vi "ConvertEdgesToLines.vi"(8 "HomeXY(pixels)":cluster{dbl, dbl}, 9 "PixelmmRatio":dbl format="%#_13g", 10 "Horizontal Edges":T1(array[cluster]) {"Point2 (Real-World)"."Y" format="%.2f"; "Point2 (Real-World)"."X" format="%.2f"; "Point1 (Real-World)"."Y" format="%.2f"; "Point1 (Real-World)"."X" format="%.2f"; "Point2 (Pixels)"."Y" format="%.2f"; "Point2 (Pixels)"."X" format="%.2f"; "Point1 (Pixels)"."Y" format="%.2f"; "Point1 (Pixels)"."X" format="%.2f"}, 11 "Vertical Edges":T1(array[cluster]) {"Point2 (Real-World)"."Y" format="%.2f"; "Point2 (Real-World)"."X" format="%.2f"; "Point1 (Real-World)"."Y" format="%.2f"; "Point1 (Real-World)"."X" format="%.2f"; "Point2 (Pixels)"."Y" format="%.2f"; "Point2 (Pixels)"."X" format="%.2f"; "Point1 (Pixels)"."Y" format="%.2f"; "Point1 (Pixels)"."X" format="%.2f"}) -> (1 "Lw Right":dbl[](array[numeric]), 2 "Lw Left":dbl[](array[numeric]), 3 "Lg":dbl[](array[numeric]))   [LabVIEW 2017]
uses:
  <vilib>/vision/NI_Vision_Development_Module.lvlib
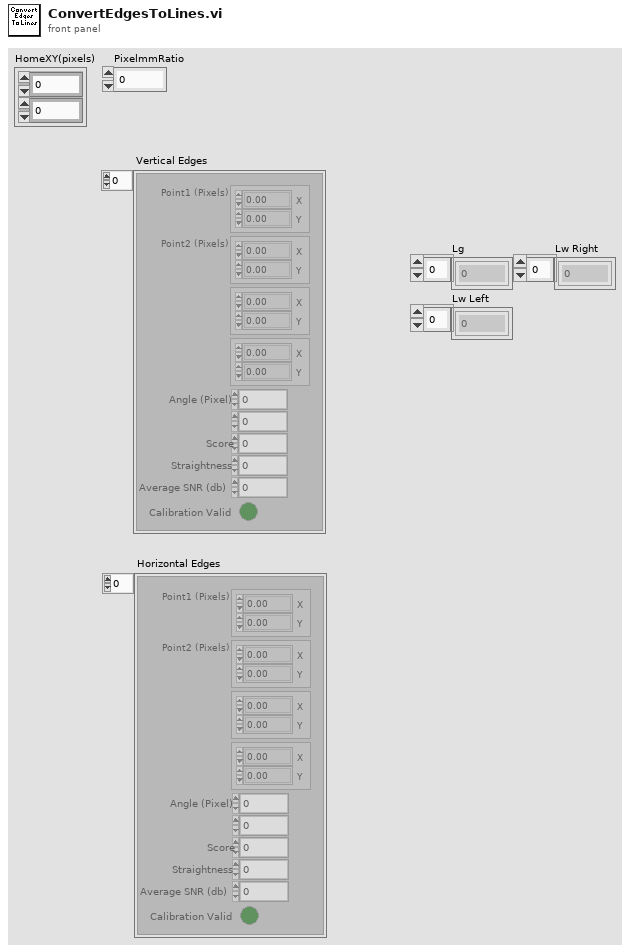
[diagram p1: front panel]
types:
  T1 = cluster{"Point1 (Pixels)":cluster{"X":sgl, "Y":sgl}, "Point2 (Pixels)":cluster{"X":sgl, "Y":sgl}, "Point1 (Real-World)":cluster{"X":sgl, "Y":sgl}, "Point2 (Real-World)":cluster{"X":sgl, "Y":sgl}, "Angle (Pixel)":dbl, "Angle (Real-World)":dbl, "Score":dbl, "Straightness":dbl, "Average SNR (db)":dbl, "Calibration Valid":bool}[]
  T2 = cluster{"Vertical Edges[0]":cluster{"Point1 (Pixels)":cluster{"X":sgl, "Y":sgl}, "Point2 (Pixels)":cluster{"X":sgl, "Y":sgl}, "Point1 (Real-World)":cluster{"X":sgl, "Y":sgl}, "Point2 (Real-World)":cluster{"X":sgl, "Y":sgl}, "Angle (Pixel)":dbl, "Angle (Real-World)":dbl, "Score":dbl, "Straightness":dbl, "Average SNR (db)":dbl, "Calibration Valid":bool}, "Vertical Edges[1]":cluster{"Point1 (Pixels)":cluster{"X":sgl, "Y":sgl}, "Point2 (Pixels)":cluster{"X":sgl, "Y":sgl}, "Point1 (Real-World)":cluster{"X":sgl, "Y":sgl}, "Point2 (Real-World)":cluster{"X":sgl, "Y":sgl}, "Angle (Pixel)":dbl, "Angle (Real-World)":dbl, "Score":dbl, "Straightness":dbl, "Average SNR (db)":dbl, "Calibration Valid":bool}, "Vertical Edges[2]":cluster{"Point1 (Pixels)":cluster{"X":sgl, "Y":sgl}, "Point2 (Pixels)":cluster{"X":sgl, "Y":sgl}, "Point1 (Real-World)":cluster{"X":sgl, "Y":sgl}, "Point2 (Real-World)":cluster{"X":sgl, "Y":sgl}, "Angle (Pixel)":dbl, "Angle (Real-World)":dbl, "Score":dbl, "Straightness":dbl, "Average SNR (db)":dbl, "Calibration Valid":bool}, "Vertical Edges[3]":cluster{"Point1 (Pixels)":cluster{"X":sgl, "Y":sgl}, "Point2 (Pixels)":cluster{"X":sgl, "Y":sgl}, "Point1 (Real-World)":cluster{"X":sgl, "Y":sgl}, "Point2 (Real-World)":cluster{"X":sgl, "Y":sgl}, "Angle (Pixel)":dbl, "Angle (Real-World)":dbl, "Score":dbl, "Straightness":dbl, "Average SNR (db)":dbl, "Calibration Valid":bool}, "Vertical Edges[4]":cluster{"Point1 (Pixels)":cluster{"X":sgl, "Y":sgl}, "Point2 (Pixels)":cluster{"X":sgl, "Y":sgl}, "Point1 (Real-World)":cluster{"X":sgl, "Y":sgl}, "Point2 (Real-World)":cluster{"X":sgl, "Y":sgl}, "Angle (Pixel)":dbl, "Angle (Real-World)":dbl, "Score":dbl, "Straightness":dbl, "Average SNR (db)":dbl, "Calibration Valid":bool}, "Vertical Edges[5]":cluster{"Point1 (Pixels)":cluster{"X":sgl, "Y":sgl}, "Point2 (Pixels)":cluster{"X":sgl, "Y":sgl}, "Point1 (Real-World)":cluster{"X":sgl, "Y":sgl}, "Point2 (Real-World)":cluster{"X":sgl, "Y":sgl}, "Angle (Pixel)":dbl, "Angle (Real-World)":dbl, "Score":dbl, "Straightness":dbl, "Average SNR (db)":dbl, "Calibration Valid":bool}, "Vertical Edges[6]":cluster{"Point1 (Pixels)":cluster{"X":sgl, "Y":sgl}, "Point2 (Pixels)":cluster{"X":sgl, "Y":sgl}, "Point1 (Real-World)":cluster{"X":sgl, "Y":sgl}, "Point2 (Real-World)":cluster{"X":sgl, "Y":sgl}, "Angle (Pixel)":dbl, "Angle (Real-World)":dbl, "Score":dbl, "Straightness":dbl, "Average SNR (db)":dbl, "Calibration Valid":bool}, "Vertical Edges[7]":cluster{"Point1 (Pixels)":cluster{"X":sgl, "Y":sgl}, "Point2 (Pixels)":cluster{"X":sgl, "Y":sgl}, "Point1 (Real-World)":cluster{"X":sgl, "Y":sgl}, "Point2 (Real-World)":cluster{"X":sgl, "Y":sgl}, "Angle (Pixel)":dbl, "Angle (Real-World)":dbl, "Score":dbl, "Straightness":dbl, "Average SNR (db)":dbl, "Calibration Valid":bool}, "Vertical Edges[8]":cluster{"Point1 (Pixels)":cluster{"X":sgl, "Y":sgl}, "Point2 (Pixels)":cluster{"X":sgl, "Y":sgl}, "Point1 (Real-World)":cluster{"X":sgl, "Y":sgl}, "Point2 (Real-World)":cluster{"X":sgl, "Y":sgl}, "Angle (Pixel)":dbl, "Angle (Real-World)":dbl, "Score":dbl, "Straightness":dbl, "Average SNR (db)":dbl, "Calibration Valid":bool}}
  T3 = cluster{"Horizontal Edges[0]":cluster{"Point1 (Pixels)":cluster{"X":sgl, "Y":sgl}, "Point2 (Pixels)":cluster{"X":sgl, "Y":sgl}, "Point1 (Real-World)":cluster{"X":sgl, "Y":sgl}, "Point2 (Real-World)":cluster{"X":sgl, "Y":sgl}, "Angle (Pixel)":dbl, "Angle (Real-World)":dbl, "Score":dbl, "Straightness":dbl, "Average SNR (db)":dbl, "Calibration Valid":bool}, "Horizontal Edges[1]":cluster{"Point1 (Pixels)":cluster{"X":sgl, "Y":sgl}, "Point2 (Pixels)":cluster{"X":sgl, "Y":sgl}, "Point1 (Real-World)":cluster{"X":sgl, "Y":sgl}, "Point2 (Real-World)":cluster{"X":sgl, "Y":sgl}, "Angle (Pixel)":dbl, "Angle (Real-World)":dbl, "Score":dbl, "Straightness":dbl, "Average SNR (db)":dbl, "Calibration Valid":bool}, "Horizontal Edges[2]":cluster{"Point1 (Pixels)":cluster{"X":sgl, "Y":sgl}, "Point2 (Pixels)":cluster{"X":sgl, "Y":sgl}, "Point1 (Real-World)":cluster{"X":sgl, "Y":sgl}, "Point2 (Real-World)":cluster{"X":sgl, "Y":sgl}, "Angle (Pixel)":dbl, "Angle (Real-World)":dbl, "Score":dbl, "Straightness":dbl, "Average SNR (db)":dbl, "Calibration Valid":bool}, "Horizontal Edges[3]":cluster{"Point1 (Pixels)":cluster{"X":sgl, "Y":sgl}, "Point2 (Pixels)":cluster{"X":sgl, "Y":sgl}, "Point1 (Real-World)":cluster{"X":sgl, "Y":sgl}, "Point2 (Real-World)":cluster{"X":sgl, "Y":sgl}, "Angle (Pixel)":dbl, "Angle (Real-World)":dbl, "Score":dbl, "Straightness":dbl, "Average SNR (db)":dbl, "Calibration Valid":bool}, "Horizontal Edges[4]":cluster{"Point1 (Pixels)":cluster{"X":sgl, "Y":sgl}, "Point2 (Pixels)":cluster{"X":sgl, "Y":sgl}, "Point1 (Real-World)":cluster{"X":sgl, "Y":sgl}, "Point2 (Real-World)":cluster{"X":sgl, "Y":sgl}, "Angle (Pixel)":dbl, "Angle (Real-World)":dbl, "Score":dbl, "Straightness":dbl, "Average SNR (db)":dbl, "Calibration Valid":bool}, "Horizontal Edges[5]":cluster{"Point1 (Pixels)":cluster{"X":sgl, "Y":sgl}, "Point2 (Pixels)":cluster{"X":sgl, "Y":sgl}, "Point1 (Real-World)":cluster{"X":sgl, "Y":sgl}, "Point2 (Real-World)":cluster{"X":sgl, "Y":sgl}, "Angle (Pixel)":dbl, "Angle (Real-World)":dbl, "Score":dbl, "Straightness":dbl, "Average SNR (db)":dbl, "Calibration Valid":bool}, "Horizontal Edges[6]":cluster{"Point1 (Pixels)":cluster{"X":sgl, "Y":sgl}, "Point2 (Pixels)":cluster{"X":sgl, "Y":sgl}, "Point1 (Real-World)":cluster{"X":sgl, "Y":sgl}, "Point2 (Real-World)":cluster{"X":sgl, "Y":sgl}, "Angle (Pixel)":dbl, "Angle (Real-World)":dbl, "Score":dbl, "Straightness":dbl, "Average SNR (db)":dbl, "Calibration Valid":bool}, "Horizontal Edges[7]":cluster{"Point1 (Pixels)":cluster{"X":sgl, "Y":sgl}, "Point2 (Pixels)":cluster{"X":sgl, "Y":sgl}, "Point1 (Real-World)":cluster{"X":sgl, "Y":sgl}, "Point2 (Real-World)":cluster{"X":sgl, "Y":sgl}, "Angle (Pixel)":dbl, "Angle (Real-World)":dbl, "Score":dbl, "Straightness":dbl, "Average SNR (db)":dbl, "Calibration Valid":bool}, "Horizontal Edges[8]":cluster{"Point1 (Pixels)":cluster{"X":sgl, "Y":sgl}, "Point2 (Pixels)":cluster{"X":sgl, "Y":sgl}, "Point1 (Real-World)":cluster{"X":sgl, "Y":sgl}, "Point2 (Real-World)":cluster{"X":sgl, "Y":sgl}, "Angle (Pixel)":dbl, "Angle (Real-World)":dbl, "Score":dbl, "Straightness":dbl, "Average SNR (db)":dbl, "Calibration Valid":bool}}
  T4 = cluster{"Point1 (Pixels)":cluster{"X":sgl, "Y":sgl}, "Point2 (Pixels)":cluster{"X":sgl, "Y":sgl}, "Point1 (Real-World)":cluster{"X":sgl, "Y":sgl}, "Point2 (Real-World)":cluster{"X":sgl, "Y":sgl}, "Angle (Pixel)":dbl, "Angle (Real-World)":dbl, "Score":dbl, "Straightness":dbl, "Average SNR (db)":dbl, "Calibration Valid":bool}
  T5 = cluster{"Point1 (Real-World)":cluster{"X":sgl, "Y":sgl}, "Point2 (Real-World)":cluster{"X":sgl, "Y":sgl}}
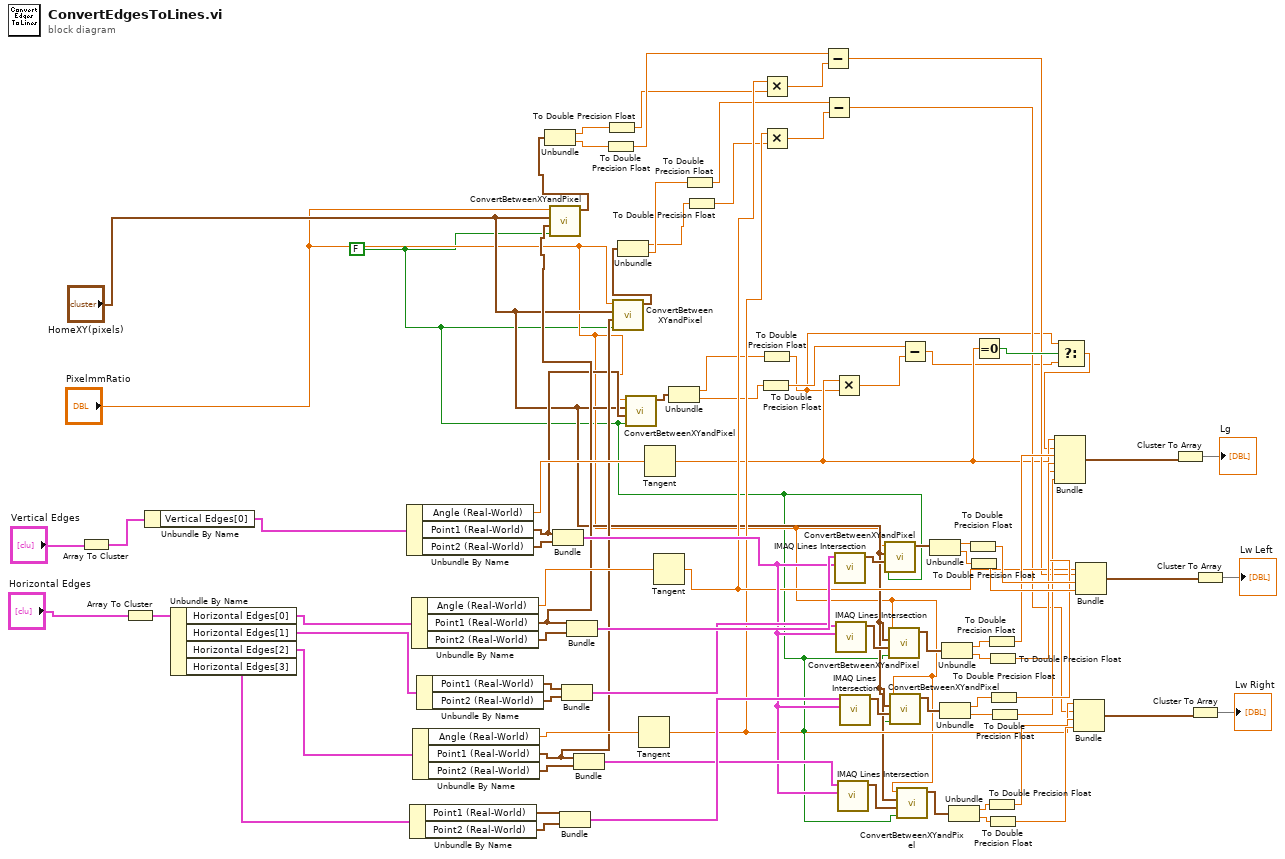
[diagram p0: block diagram]
diagram:
  w1 = FALSE ("XYtoPixels")
  n1 = Array To Cluster(array="Vertical Edges") -> (cluster=w85:T2)
  n2 = Array To Cluster(array="Horizontal Edges") -> (cluster=w83:T3)
  n3 = Unbundle By Name(w85) -> ("Vertical Edges[0]"=w77:T4)
  n4 = Unbundle By Name(w83) -> ("Horizontal Edges[0]"=w82:T4, "Horizontal Edges[1]"=w79:T4, "Horizontal Edges[2]"=w80:T4, "Horizontal Edges[3]"=w78:T4)
  n5 = Unbundle By Name(w77) -> ("Angle (Real-World)"=w68:dbl, "Point1 (Real-World)"=w7:cluster{"X":sgl, "Y":sgl}, "Point2 (Real-World)"=w75:cluster{"X":sgl, "Y":sgl})
  n6 = Unbundle By Name(w78) -> ("Point1 (Real-World)"=w72:cluster{"X":sgl, "Y":sgl}, "Point2 (Real-World)"=w71:cluster{"X":sgl, "Y":sgl})
  n7 = Unbundle By Name(w82) -> ("Angle (Real-World)"=w69:dbl, "Point1 (Real-World)"=w31:cluster{"X":sgl, "Y":sgl}, "Point2 (Real-World)"=w81:cluster{"X":sgl, "Y":sgl})
  n8 = Unbundle By Name(w80) -> ("Angle (Real-World)"=w70:dbl, "Point1 (Real-World)"=w27:cluster{"X":sgl, "Y":sgl}, "Point2 (Real-World)"=w76:cluster{"X":sgl, "Y":sgl})
  n9 = Unbundle By Name(w79) -> ("Point1 (Real-World)"=w74:cluster{"X":sgl, "Y":sgl}, "Point2 (Real-World)"=w73:cluster{"X":sgl, "Y":sgl})
  n10 = call "ConvertBetweenXYandPixel.vi"("XYtoPixels"=w1, "PointToConvert"=w31, "HomeXY(pixels)"="HomeXY(pixels)", "Pixel/mm"="PixelmmRatio") -> ("Point"=w30:cluster{sgl, sgl})  [unwired: 7 in]
  n11 = Unbundle(w30) -> (w29:sgl, w28:sgl)
  n12 = Bundle("Point1 (Real-World)"=w7, "Point2 (Real-World)"=w75) -> (w61:T5)  [unwired: 1 in]
  n13 = Bundle("Point1 (Real-World)"=w72, "Point2 (Real-World)"=w71) -> (w63:T5)  [unwired: 1 in]
  n14 = Bundle("Point1 (Real-World)"=w74, "Point2 (Real-World)"=w73) -> (w64:T5)  [unwired: 1 in]
  n15 = Bundle("Point1 (Real-World)"=w31, "Point2 (Real-World)"=w81) -> (w67:T5)  [unwired: 1 in]
  n16 = Bundle("Point1 (Real-World)"=w27, "Point2 (Real-World)"=w76) -> (w62:T5)  [unwired: 1 in]
  n17 = To Double Precision Float(number=w28) -> (double precision float=w49:dbl)
  n18 = To Double Precision Float(number=w29) -> (double precision float=w47:dbl)
  n19 = call "ConvertBetweenXYandPixel.vi"("XYtoPixels"=w1, "PointToConvert"=w27, "HomeXY(pixels)"="HomeXY(pixels)", "Pixel/mm"="PixelmmRatio") -> ("Point"=w26:cluster{sgl, sgl})  [unwired: 7 in]
  n20 = Unbundle(w26) -> (w24:sgl, w25:sgl)
  n21 = call "ConvertBetweenXYandPixel.vi"("XYtoPixels"=w1, "PointToConvert"=w7, "HomeXY(pixels)"="HomeXY(pixels)", "Pixel/mm"="PixelmmRatio") -> ("Point"=w6:cluster{sgl, sgl})  [unwired: 7 in]
  n22 = Tangent(1:w70) -> (0:w52:dbl)
  n23 = Tangent(1:w68) -> (0:w36:dbl)
  n24 = Tangent(1:w69) -> (0:w53:dbl)
  n25 = Unbundle(w6) -> (w5:sgl, w4:sgl)
  n26 = To Double Precision Float(number=w25) -> (double precision float=w48:dbl)
  n27 = To Double Precision Float(number=w24) -> (double precision float=w46:dbl)
  n28 = To Double Precision Float(number=w4) -> (double precision float=w45:dbl)
  n29 = Multiply(x=w53, y=w47) -> (x*y=w51:dbl)
  n30 = Multiply(x=w52, y=w46) -> (x*y=w50:dbl)
  n31 = To Double Precision Float(number=w5) -> (double precision float=w35:dbl)
  n32 = Subtract(x=w49, y=w51) -> (x-y=w38:dbl)
  n33 = Subtract(x=w48, y=w50) -> (x-y=w37:dbl)
  n34 = Multiply(x=w36, y=w35) -> (x*y=w44:dbl)
  n35 = call "IMAQ Lines Intersection"("Line 2"=w61, "Line 1"=w67) -> ("Intersection Point"=w20:cluster{"X":sgl, "Y":sgl})  [unwired: 7 in, 2 out]
  n36 = call "IMAQ Lines Intersection"("Line 2"=w61, "Line 1"=w64) -> ("Intersection Point"=w19:cluster{"X":sgl, "Y":sgl})  [unwired: 7 in, 2 out]
  n37 = call "IMAQ Lines Intersection"("Line 2"=w61, "Line 1"=w62) -> ("Intersection Point"=w17:cluster{"X":sgl, "Y":sgl})  [unwired: 7 in, 2 out]
  n38 = call "IMAQ Lines Intersection"("Line 2"=w61, "Line 1"=w63) -> ("Intersection Point"=w18:cluster{"X":sgl, "Y":sgl})  [unwired: 7 in, 2 out]
  n39 = call "ConvertBetweenXYandPixel.vi"("XYtoPixels"=w1, "PointToConvert"=w20, "HomeXY(pixels)"="HomeXY(pixels)", "Pixel/mm"="PixelmmRatio") -> ("Point"=w23:cluster{sgl, sgl})  [unwired: 7 in]
  n40 = call "ConvertBetweenXYandPixel.vi"("XYtoPixels"=w1, "PointToConvert"=w19, "HomeXY(pixels)"="HomeXY(pixels)", "Pixel/mm"="PixelmmRatio") -> ("Point"=w14:cluster{sgl, sgl})  [unwired: 7 in]
  n41 = call "ConvertBetweenXYandPixel.vi"("XYtoPixels"=w1, "PointToConvert"=w18, "HomeXY(pixels)"="HomeXY(pixels)", "Pixel/mm"="PixelmmRatio") -> ("Point"=w15:cluster{sgl, sgl})  [unwired: 7 in]
  n42 = call "ConvertBetweenXYandPixel.vi"("XYtoPixels"=w1, "PointToConvert"=w17, "HomeXY(pixels)"="HomeXY(pixels)", "Pixel/mm"="PixelmmRatio") -> ("Point"=w16:cluster{sgl, sgl})  [unwired: 7 in]
  n43 = Subtract(x=w45, y=w44) -> (x-y=w34:dbl)
  n44 = Unbundle(w23) -> (w22:sgl, w21:sgl)
  n45 = Unbundle(w15) -> (w11:sgl, w10:sgl)
  n46 = Unbundle(w14) -> (w13:sgl, w12:sgl)
  n47 = Unbundle(w16) -> (w9:sgl, w8:sgl)
  n48 = To Double Precision Float(number=w22) -> (double precision float=w66:dbl)
  n49 = To Double Precision Float(number=w21) -> (double precision float=w65:dbl)
  n50 = Equal To 0?(x=w36) -> (x = 0?=w54:bool)
  n51 = To Double Precision Float(number=w13) -> (double precision float=w60:dbl)
  n52 = To Double Precision Float(number=w9) -> (double precision float=w56:dbl)
  n53 = To Double Precision Float(number=w12) -> (double precision float=w59:dbl)
  n54 = To Double Precision Float(number=w8) -> (double precision float=w55:dbl)
  n55 = To Double Precision Float(number=w11) -> (double precision float=w58:dbl)
  n56 = To Double Precision Float(number=w10) -> (double precision float=w57:dbl)
  n57 = Select(t=w35, s=w54, f=w34) -> (s? t:f=w33:dbl)
  n58 = Bundle(w36, w33, w60, w59, w58, w57) -> (w43:cluster{dbl, dbl, dbl, dbl, dbl, dbl})  [unwired: 1 in]
  n59 = Bundle(w52, w37, w56, w55) -> (w32:cluster{dbl, dbl, dbl, dbl})  [unwired: 1 in]
  n60 = Bundle(w53, w38, w66, w65) -> (w42:cluster{dbl, dbl, dbl, dbl})  [unwired: 1 in]
  n61 = Cluster To Array(cluster=w43) -> (array=→"Lg":dbl[])
  n62 = Cluster To Array(cluster=w32) -> (array=→"Lw Right":dbl[])
  n63 = Cluster To Array(cluster=w42) -> (array=→"Lw Left":dbl[])
